vi "Variant_Set_TS_Propss_Array_LV2015.vi"(8 "error in (no error)":errorcluster, 9 "newValue":variant, 10 "lookupString":string, 11 "Automation Refnum in":refnum<k7>) -> (0 "error out":errorcluster, 3 "reference out":refnum<k7>)   [LabVIEW 2015]
panel:
  # "Connector Pane"
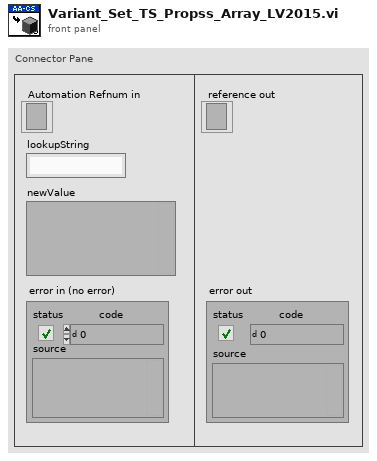
[diagram p1: front panel]
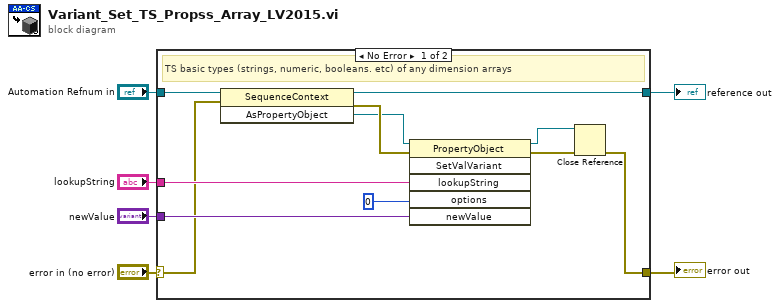
[diagram p0: block diagram]
diagram:
  n1 = case shown="No Error" "error in (no error)" {
    selector: "error in (no error)" -> [w8 w19]
    tunnel: "lookupString" -> [w17 _]
    tunnel: "Automation Refnum in" -> [w16 w18]
    tunnel: "newValue" -> [w11 _]
    tunnel: [w9 w19] -> w3
    tunnel: [w7 w18] -> w1
    frame No Error {
      # "TS basic types (strings, numeric, booleans. etc) of any dimension arrays"
      n2 = invoke class="SequenceContext" method="AsPropertyObject"(reference=w16, error in=w8) -> (reference out=w7:refnum<k7>, error out=w15:errorcluster, "AsPropertyObject"=w12:refnum<k7>)  [unwired: 1 in]
      n3 = invoke class="PropertyObject" method="SetValVariant"(reference=w12, error in=w15, "lookupString"=w17, "options"=0, "newValue"=w11) -> (reference out=w13:refnum<k7>, error out=w14:errorcluster)  [unwired: 1 in, 4 out]
      n4 = Close Reference(reference=w13, error in (no error)=w14) -> (error out=w9:errorcluster)
    }
    frame Error {
    }
  }
  "error out" <- w3
  "reference out" <- w1
